vi "redLocation.vi"() -> (0 "range":string, 1 "pos":string, 2 "Dataout":string="b")   [LabVIEW 2017]
panel:
  out "Image Out":T1(plugin-control)
  out "RED":T2
  out "size":i32
  out "Red-Data":dbl[](array[numeric])
  out "convex hull area":dbl
  out "Tayang":dbl
  out "Area":dbl
  out "Height":dbl
  out "Width":dbl
  out "Bottom":dbl
  out "Right":dbl
  out "Up":dbl
  out "Left":dbl
  out "CenterY":dbl
  out "CenterX":dbl
  out "Numeric":i32
  out "red_stop":bool
  out "Number of Particles":i32
  # "center x"
  # "center y"
  # "left"
  # "up"
  # "right"
  # "bot"
  # "width"
  # "height"
  # "tayang"
  # "area"
  # "convex hull area"
  # "img area"
  # "%area/img area"
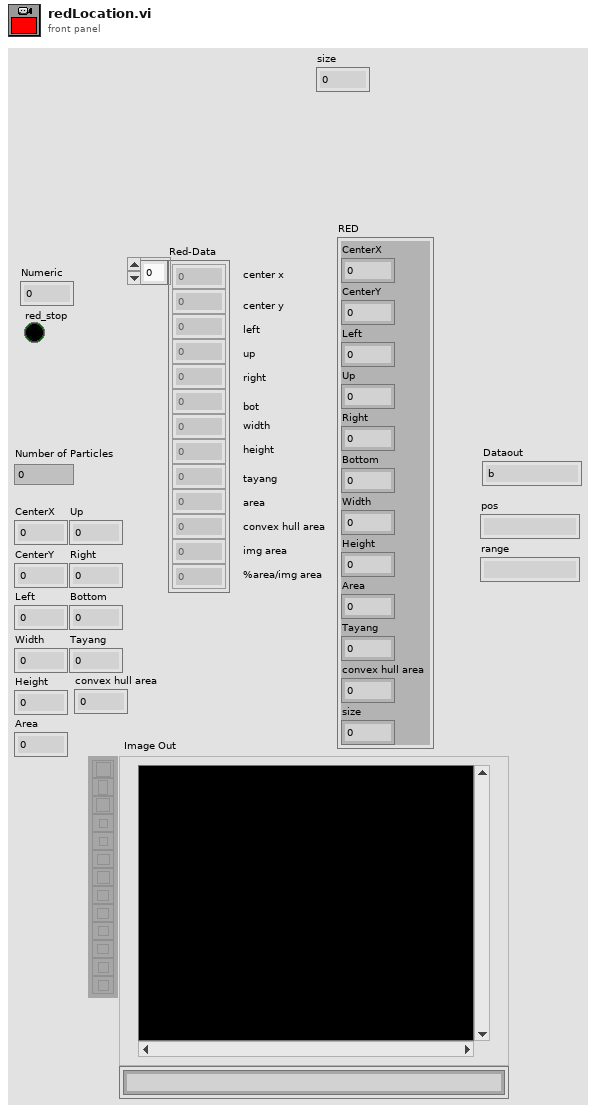
[diagram p1: front panel]
types:
  T1 = typedef "IMAQ Image.ctl" = refnum<image>
  T2 = cluster{"CenterX":dbl, "CenterY":dbl, "Left":dbl, "Up":dbl, "Right":dbl, "Bottom":dbl, "Width":dbl, "Height":dbl, "Area":dbl, "Tayang":dbl, "convex hull area":dbl, "size":i32}
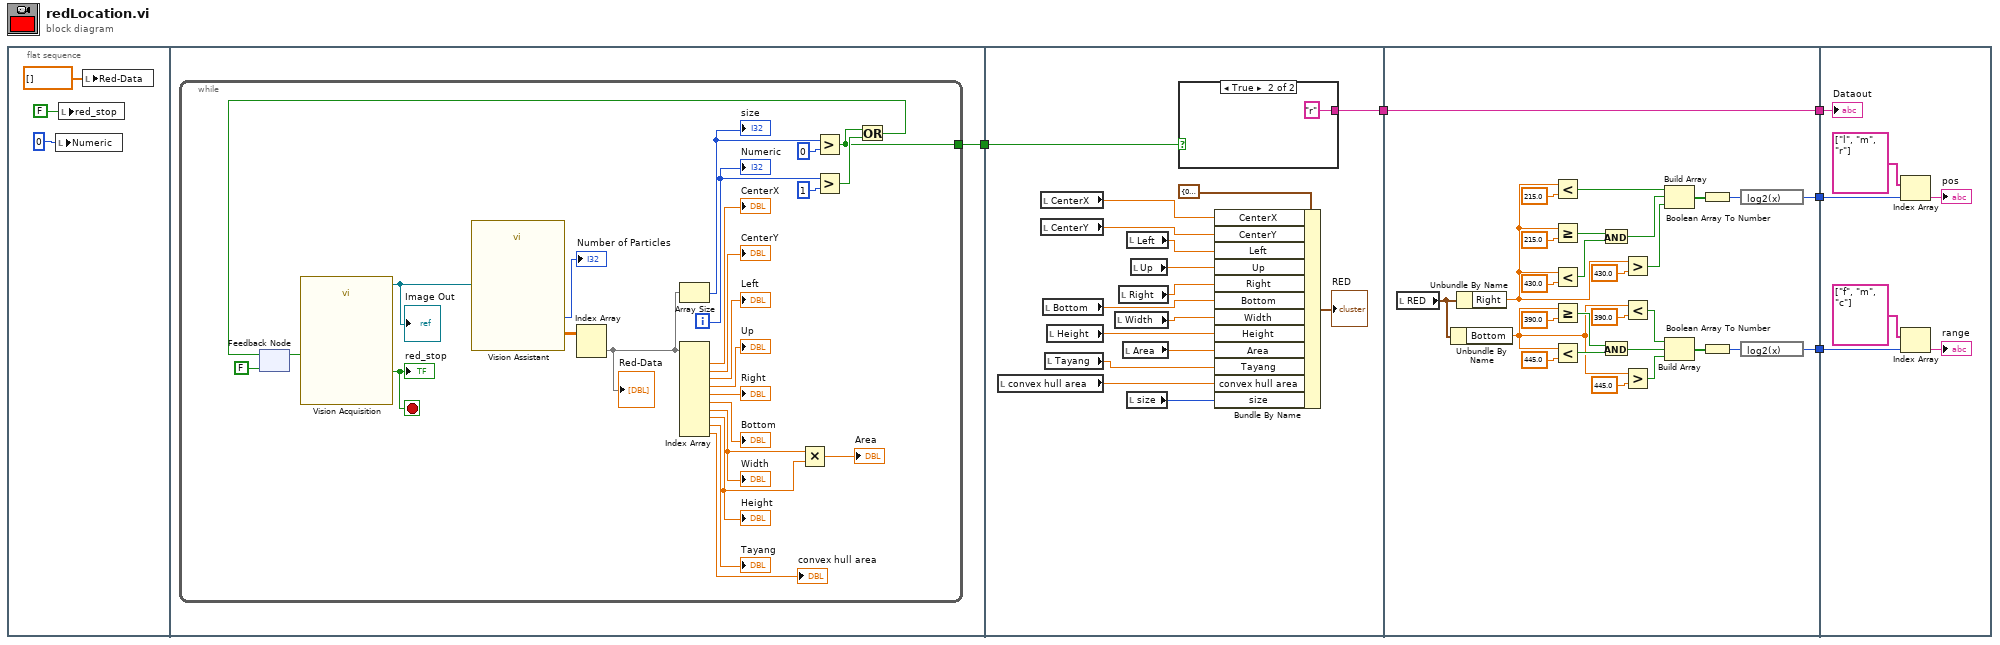
[diagram p0: block diagram]
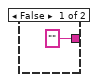
[diagram p2: hidden frame]
diagram:
  n1 = flat-sequence {
    tunnel: [w9] -> w5
    tunnel: w5 -> [w36]
    tunnel: [w35] -> w3
    tunnel: [w80] -> w4
    tunnel: w3 -> [w80]
    tunnel: [w54] -> w2
    tunnel: [w53] -> w1
    tunnel: w4 -> [w87]
    tunnel: w2 -> [w82]
    tunnel: w1 -> [w81]
    frame #0 {
      n2 = local write "Numeric"(0 ("Numeric")) -> ()
      n3 = local write "red_stop"(FALSE ("red_stop")) -> ()
      n4 = local write "Red-Data"(dbl[] [] ("Red_Data")) -> ()
    }
    frame #1 {
      n5 = while {
        tunnel: [w10] -> w9
        i -> [w28]
        stop <- w23 stop-if-true
        n6 = feedback #1(FALSE) -> (w25:bool)
        n7 = call "Vision Acquisition"("Stop (F)"=w25) -> ("Image Out"=w32:T1, "Stopped"=w23:bool)  [unwired: 24 in, 1 out]
        "red_stop" <- w23
        "Image Out" <- w32
        n8 = call "Vision Assistant"("Image In"=w32) -> ("Number of Particles (Particle Analysis 1)"=→"Number of Particles":i32, "Particle Measurements (Pixels) (Particle Analysis 1)"=w33:dbl[][])  [unwired: 23 in, 2 out]
        n9 = Index Array(array=w33) -> (element=w22:dbl[])  [unwired: 2 in]
        "Red-Data" <- w22
        n10 = Array Size(array=w22) -> (size(s)=w31:i32)
        "size" <- w31
        n11 = Index Array(array=w22) -> (element #1=→"CenterX":dbl, element #2=→"CenterY":dbl, element #3=→"Left":dbl, element #4=→"Up":dbl, element #5=→"Right":dbl, element #6=→"Bottom":dbl, element #7=w21:dbl, element #8=w20:dbl, element #9=→"Tayang":dbl, element #10=→"convex hull area":dbl)  [unwired: 10 in]
        "Width" <- w21
        "Height" <- w20
        n12 = Multiply(x=w21, y=w20) -> (x*y=→"Area":dbl)
        n13 = Greater?(x=w31, y=0) -> (0:w10:bool)
        n14 = Greater?(x=w28, y=1) -> (0:w27:bool)
        n15 = Or(x=w10, y=w27) -> (x .or. y?=w26:bool)
        n16 = feedback-in #1(w26) -> ()
        "Numeric" <- w28
      }
    }
    frame #2 {
      n17 = local read "convex hull area"() -> (w40:dbl)
      n18 = local read "CenterX"() -> (w50:dbl)
      n19 = local read "CenterY"() -> (w49:dbl)
      n20 = local read "Bottom"() -> (w45:dbl)
      n21 = local read "Tayang"() -> (w41:dbl)
      n22 = local read "Height"() -> (w43:dbl)
      n23 = local read "Width"() -> (w44:dbl)
      n24 = local read "Right"() -> (w46:dbl)
      n25 = local read "Area"() -> (w42:dbl)
      n26 = local read "Left"() -> (w48:dbl)
      n27 = local read "size"() -> (w38:i32)
      n28 = local read "Up"() -> (w47:dbl)
      n29 = case shown="True" w36 {
        tunnel: ["" "r"] -> w35
        frame False {
        }
        frame True {
        }
      }
      n30 = Bundle By Name(cluster=T2 {"CenterX"=0.0, "CenterY"=0.0, "Left"=0.0, "Up"=0.0, "Right"=0.0, "Bottom"=0.0, "Width"=0.0, "Height"=0.0, "Area"=0.0, "Tayang"=0.0, "convex hull area"=0.0, "size"=0} ("output cluster"), "CenterX"=w50, "CenterY"=w49, "Left"=w48, "Up"=w47, "Right"=w46, "Bottom"=w45, "Width"=w44, "Height"=w43, "Area"=w42, "Tayang"=w41, "convex hull area"=w40, "size"=w38) -> (→"RED":T2)
    }
    frame #3 {
      n31 = local read "RED"() -> (w55:T2)
      n32 = Unbundle By Name(w55) -> ("Bottom"=w57:dbl)
      n33 = Unbundle By Name(w55) -> ("Right"=w56:dbl)
      n34 = Less?(x=w56, y=215.0) -> (x < y?=w73:bool)
      n35 = Greater Or Equal?(x=w56, y=215.0) -> (x >= y?=w76:bool)
      n36 = Less?(x=w56, y=430.0) -> (x < y?=w75:bool)
      n37 = Greater Or Equal?(x=w57, y=390.0) -> (x >= y?=w65:bool)
      n38 = Less?(x=w57, y=445.0) -> (x < y?=w64:bool)
      n39 = And(x=w76, y=w75) -> (x .and. y?=w72:bool)
      n40 = And(x=w65, y=w64) -> (x .and. y?=w59:bool)
      n41 = Greater?(x=w56, y=430.0) -> (0:w71:bool)
      n42 = Less?(x=w57, y=390.0) -> (x < y?=w60:bool)
      n43 = Greater?(x=w57, y=445.0) -> (0:w58:bool)
      n44 = Build Array(w73, w72, w71) -> (w70:bool[])
      n45 = Build Array(w60, w59, w58) -> (w62:bool[])
      n46 = Boolean Array To Number(Boolean array=w70) -> (number=w69:u32)
      n47 = Boolean Array To Number(Boolean array=w62) -> (number=w61:u32)
      n48 = expression code="log2(x)"(w69) -> (w53:u32)
      n49 = expression code="log2(x)"(w61) -> (w54:u32)
    }
    frame #4 {
      n50 = Index Array(array=string[] ["l", "m", "r"], index=w81) -> (element=→"pos":string)
      n51 = Index Array(array=string[] ["f", "m", "c"], index=w82) -> (element=→"range":string)
      "Dataout" <- w87
    }
  }
